vi "plainPaint.vi"(7 "colourSpec":cluster{"colour":u32, "Alpha":sgl}={"colour"=0, "Alpha"=0.95} {"Alpha" min=0.2 max=1 step=0.02}, 8 "error in (no error)":errorcluster, 11 "reference":refnum<vi>) -> (0 "error out":errorcluster, 3 "reference out":refnum<vi>)   [LabVIEW 2022 SP3]
uses:
  <vilib>/Utility/miscctls.llb/LVRGBAColorTypeDef.ctl
  <vilib>/picture/3D Picture Control/NI_3D Picture Control.lvlib
panel:
  in  "Material:Color Mode":T1(ring)
  in  "Blending:Mode":enum16{"Inherit Value", "Off", "On"}(ring)=enum."On"
  in  "Blending:Function:Source":T2(ring)=enum."Source Alpha"
  in  "Blending:Function:Destination":T3(ring)=enum."One Minus Source Alpha"
  in  "Blending:Bin":T4(ring)=enum."Transparent Bin"
  in  "Specials:Anti-aliasing":enum16{"Inherit Value", "Off", "On"}(ring)=enum."On"
  in  "Specials:Shade Model":enum16{"Inherit Value", "Flat", "Smooth"}(ring)=enum."Smooth"
  in  "Specials:Lighting":enum16{"Inherit Value", "Off", "On"}(ring)=enum."On"
  in  "Specials:Autonormalizing":enum16{"Inherit Value", "Off", "On"}(ring)=enum."On"
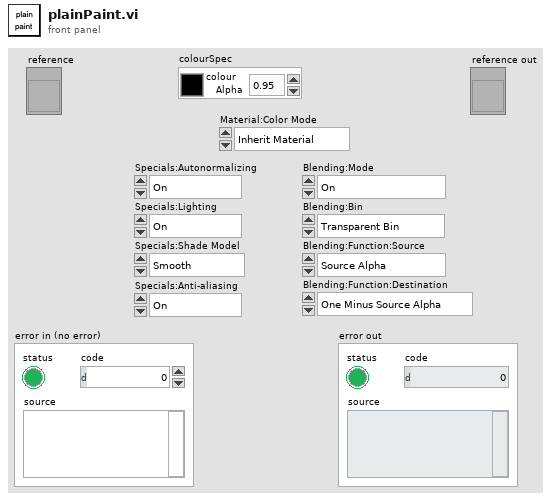
[diagram p1: front panel]
types:
  T1 = enum16{"Inherit Material", "Use entire Material", "Ignore Ambient", "Ignore Diffuse", "Ignore Specular", "Ignore Emission", "Ignore Ambient and Diffuse"}
  T2 = enum16{"Zero", "One", "Destination Color", "One Minus Destination Color", "Source Alpha", "One Minus Source Alpha", "Destination Alpha", "One Minus Destination Alpha", "Source Alpha Saturate"}
  T3 = enum16{"Zero", "One", "Source Color", "One Minus Source Color", "Source Alpha", "One Minus Source Alpha", "Destination Alpha", "One Minus Destination Alpha"}
  T4 = enum16{"Normal Bin", "Opaque Bin", "Transparent Bin"}
  T5 = typedef "LVRGBAColorTypeDef.ctl" = cluster{"Red":sgl, "Green":sgl, "Blue":sgl, "Alpha":sgl}
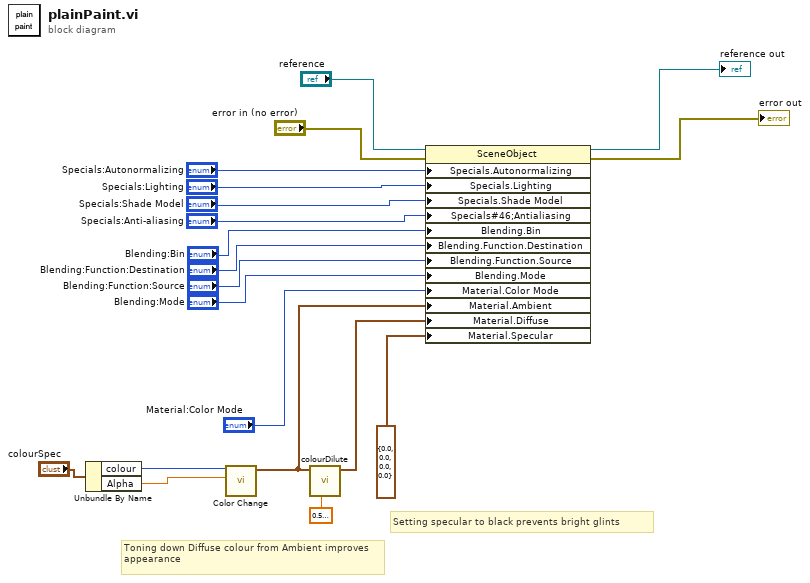
[diagram p0: block diagram]
diagram:
  # "Toning down Diffuse colour from Ambient improves appearance"
  # "Setting specular to black prevents bright glints"
  n1 = Unbundle By Name("colourSpec") -> ("colour"=w2:u32, "Alpha"=w1:sgl)
  n2 = call <vilib>:"Color Change.vi"("Alpha"=w1, "Color"=w2) -> ("RGBA"=w7:cluster{"R":sgl, "G":sgl, "B":sgl, "A":sgl})  [unwired: 9 in]
  n3 = call "colourDilute.vi"("dilutionFactor"=0.5000000000000001, "RGBIn"=w7) -> ("RGBOut"=w6:cluster{"R":dbl, "G":dbl, "B":dbl, "A":dbl})  [unwired: 8 in, 1 out]
  n4 = property class="SceneObject"(reference="reference", error in="error in (no error)", "Specials.Autonormalizing"="Specials:Autonormalizing", "Specials.Lighting"="Specials:Lighting", "Specials.Shade Model"="Specials:Shade Model", "Specials#46;Antialiasing"="Specials:Anti-aliasing", "Blending.Bin"="Blending:Bin", "Blending.Function.Destination"="Blending:Function:Destination", "Blending.Function.Source"="Blending:Function:Source", "Blending.Mode"="Blending:Mode", "Material.Color Mode"="Material:Color Mode", "Material.Ambient"=w7, "Material.Diffuse"=w6, "Material.Specular"=T5 {"Red"=0.0, "Green"=0.0, "Blue"=0.0, "Alpha"=0.0} ("Material:Specular")) -> (reference out=→"reference out":refnum<vi>, error out=→"error out":errorcluster)
